vi "DataArrangement.vi"(8 "error in (no error)":errorcluster, 9 "DataType":variant[](array[variant]), 11 "file path (dialog if empty)":path) -> (0 "error out":errorcluster, 1 "DataList":variant[](array[variant]), 3 "CmdList":string[](array[string]))   [LabVIEW 2014]
uses:
  <vilib>/Utility/file.llb/Read From Spreadsheet File (string).vi
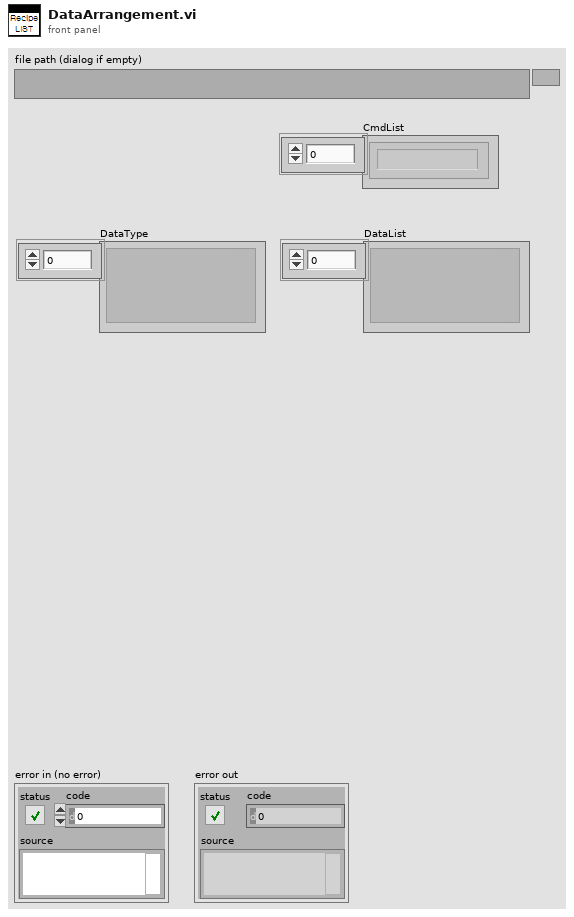
[diagram p1: front panel]
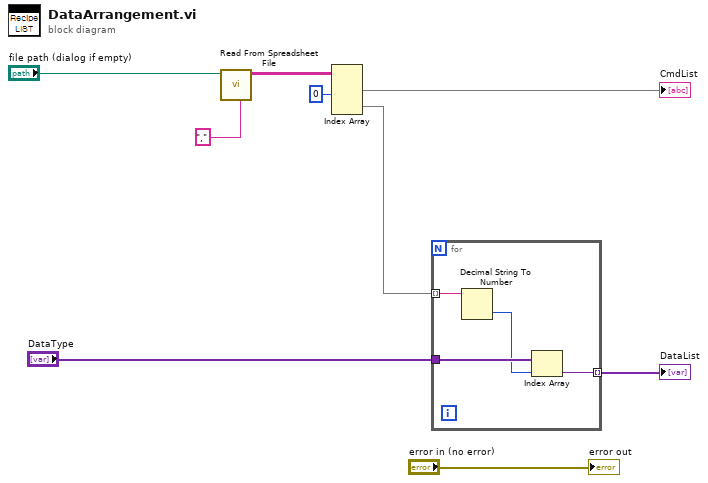
[diagram p0: block diagram]
diagram:
  n1 = call-poly <vilib>:"Read From Spreadsheet File.vi"("delimiter (\\t)"="," ("delimiter (\\t)"), "file path (dialog if empty)"="file path (dialog if empty)") -> ("all rows"=w7:string[][])  [unwired: 5 in, 4 out]
  n2 = Index Array(array=w7, index (col) #1=0 ("disabled index (col)")) -> (element #1=→"CmdList":string[], element #2=w5:string[])  [unwired: 3 in]
  n3 = for {
    tunnel: w5 -> [w13] mode=indexing
    tunnel: "DataType" -> [w12]
    tunnel: [w10] -> w3 mode=indexing
    n4 = Decimal String To Number(string=w13) -> (number=w11:i32)  [unwired: 2 in, 1 out]
    n5 = Index Array(array=w12, index=w11) -> (element=w10:variant)
  }
  "DataList" <- w3
  "error out" <- "error in (no error)"
